vi "GetProdLine.vi"(10 "Lotno":string) -> (2 "ProdLine":string)   [LabVIEW 2012]
uses:
  <vilib>/addons/database/Auxilliary.llb/DB Tools Cursor Type.ctl
  Global1.vi
  <vilib>/addons/database/Connection.llb/DB Tools Open Connec (Path).vi
  <vilib>/addons/database/Connection.llb/Conn Execute.vi
  <vilib>/addons/database/Recordset.llb/Rec Fetch Integer Data (R).vi
  <vilib>/addons/database/Recordset.llb/Rec Destroy - Connection.vi
  <vilib>/addons/database/Recordset.llb/Rec Fetch String Data (R).vi
  <vilib>/addons/database/NI_Database_API.lvlib
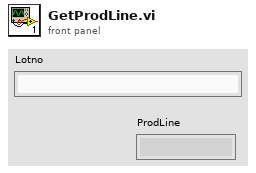
[diagram p1: front panel]
types:
  T1 = typedef "NI_Database_API.lvlib/DB Tools Cursor Type.ctl" = enum16{"forward-only", "keyset", "dynamic", "static"}
  T2 = typedef "NI_Database_API.lvlib/Conn ObjectReference.ctl" = refnum<k1>
  T3 = typedef "NI_Database_API.lvlib/Rec ObjectReference.ctl" = refnum<k1>
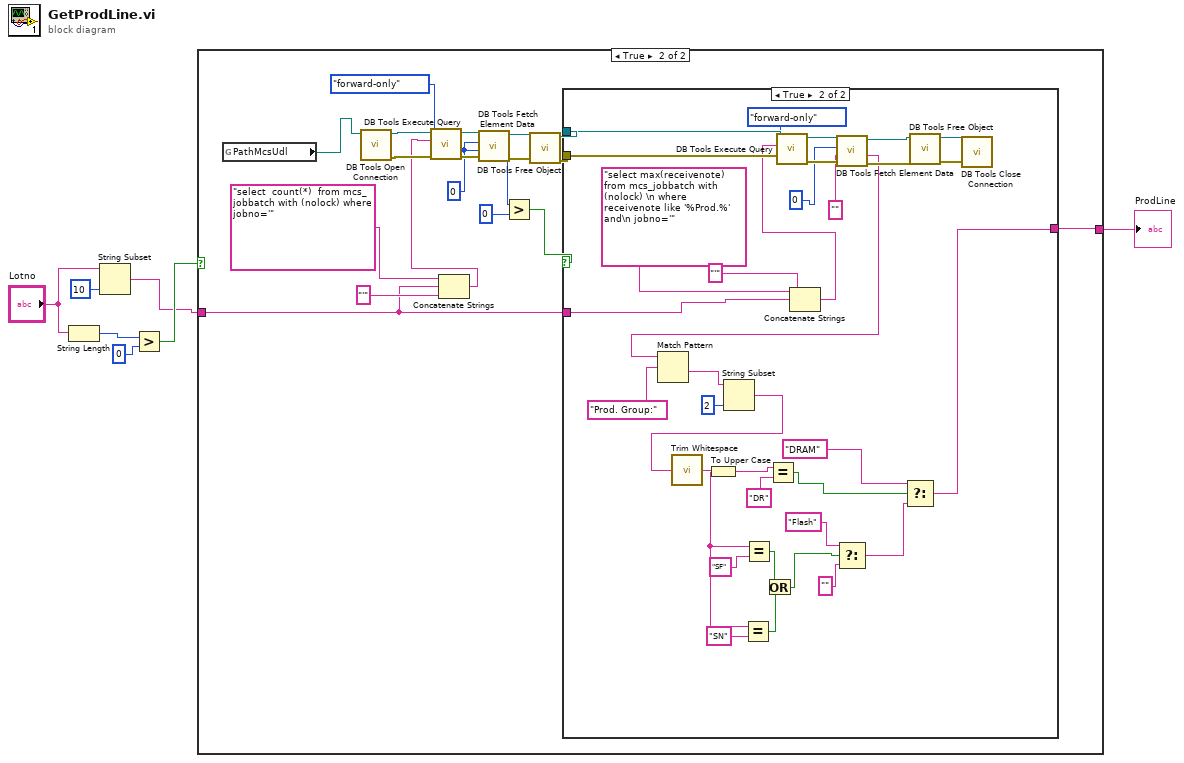
[diagram p0: block diagram]
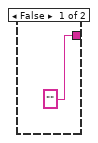
[diagram p2: hidden frame]
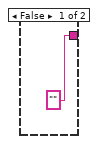
[diagram p3: hidden frame]
diagram:
  n1 = String Length(string="Lotno") -> (length=w7:i32)
  n2 = String Subset(string="Lotno", length (rest)=10 ("length (rest)")) -> (substring=w2:string)  [unwired: 1 in]
  n3 = Greater?(x=w7, y=0) -> (0:w5:bool)
  n4 = case shown="True" w5 {
    tunnel: w2 -> [_ w21]
    tunnel: ["" ("data") w9] -> w4
    frame False {
    }
    frame True {
      w14 = 0
      n5 = global read "Global1.vi" "PathMcsUdl"() -> (w10:path)
      n6 = call-poly <vilib>:"DB Tools Open Connection.vi"("connection information"=w10) -> ("error out"=w24:errorcluster, "connection reference"=w25:T2)  [unwired: 7 in]
      n7 = Concatenate Strings("select  count(*)  from mcs_jobbatch with (nolock) where jobno='" ("string"), w21, "'" ("string")) -> (w19:string)
      n8 = call-poly <vilib>:"DB Tools Execute Query.vi"("error in (no error)"=w24, "cursor type"=DB_Tools_Cursor_Type."forward-only", "SQL query"=w19, "connection reference"=w25) -> ("error out"=w18:errorcluster, "recordset reference"=w17:T3)  [unwired: 4 in]
      n9 = call-poly <vilib>:"DB Tools Fetch Element Data.vi"("error in (no error)"=w18, "type"=w14, "column index"=w14, "recordset reference"=w17) -> ("error out"=w15:errorcluster, "data"=w13:i32, "recordset reference out"=w16:T3)  [unwired: 3 in]
      n10 = Greater?(x=w13, y=0) -> (0:w11:bool)
      n11 = call-poly <vilib>:"DB Tools Free Object.vi"("error in (no error)"=w15, "recordset reference"=w16) -> ("error out"=w26:errorcluster, "connection reference"=w27:T2)  [unwired: 8 in]
      n12 = case shown="True" w11 {
        tunnel: w27 -> [_ w60]
        tunnel: w26 -> [_ w57]
        tunnel: w21 -> [_ w50]
        tunnel: ["" ("data") w37] -> w9
        frame False {
        }
        frame True {
          n13 = Concatenate Strings("select max(receivenote)  from mcs_jobbatch with (nolock) \n where receivenote like '%Prod.%' and\n jobno='" ("string"), w50, "'" ("string")) -> (w51:string)
          n14 = call-poly <vilib>:"DB Tools Execute Query.vi"("error in (no error)"=w57, "cursor type"=DB_Tools_Cursor_Type."forward-only", "SQL query"=w51, "connection reference"=w60) -> ("error out"=w56:errorcluster, "recordset reference"=w59:T3)  [unwired: 4 in]
          n15 = call-poly <vilib>:"DB Tools Fetch Element Data.vi"("error in (no error)"=w56, "type"="", "column index"=0, "recordset reference"=w59) -> ("error out"=w55:errorcluster, "data"=w47:string, "recordset reference out"=w58:T3)  [unwired: 3 in]
          n16 = Match Pattern(string=w47, regular expression="Prod. Group:") -> (after substring=w36:string)  [unwired: 1 in, 3 out]
          n17 = String Subset(string=w36, length (rest)=2 ("length (rest)")) -> (substring=w34:string)  [unwired: 1 in]
          n18 = call <vilib>:"Trim Whitespace.vi"("string"=w34) -> ("trimmed string"=w45:string)  [unwired: 1 in]
          n19 = To Upper Case(1:w45) -> (0:w33:string)
          n20 = Equal?(x=w33, y="SN") -> (x = y?=w30:bool)
          n21 = Equal?(x=w33, y="SF") -> (x = y?=w31:bool)
          n22 = Or(x=w31, y=w30) -> (x .or. y?=w29:bool)
          n23 = Equal?(x=w33, y="DR") -> (x = y?=w43:bool)
          n24 = Select(t="Flash", s=w29, f="") -> (s? t:f=w39:string)
          n25 = Select(t="DRAM", s=w43, f=w39) -> (s? t:f=w37:string)
          n26 = call-poly <vilib>:"DB Tools Free Object.vi"("error in (no error)"=w55, "recordset reference"=w58) -> ("error out"=w62:errorcluster, "connection reference"=w61:T2)  [unwired: 8 in]
          n27 = call <vilib>:"DB Tools Close Connection.vi"("error in (no error)"=w62, "connection reference"=w61) -> ()  [unwired: 5 in, 1 out]
        }
      }
    }
  }
  "ProdLine" <- w4
